vi "Disconnect All.vi"(8 "error in (no error)":errorcluster, 11 "Consumer in":refnum<class "Consumer.lvclass">) -> (0 "error out":errorcluster, 3 "Consumer out":refnum<class "Consumer.lvclass">)   [LabVIEW 2017, in "%DEVICE% Messaging.lvlib" / "Consumer.lvclass"]
uses:
  Consumer.lvclass
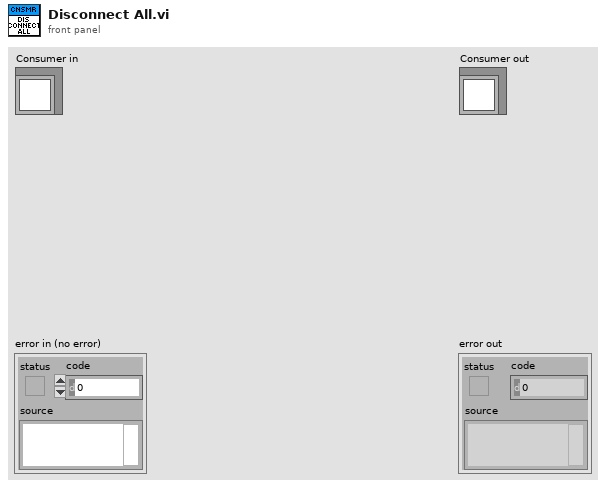
[diagram p1: front panel]
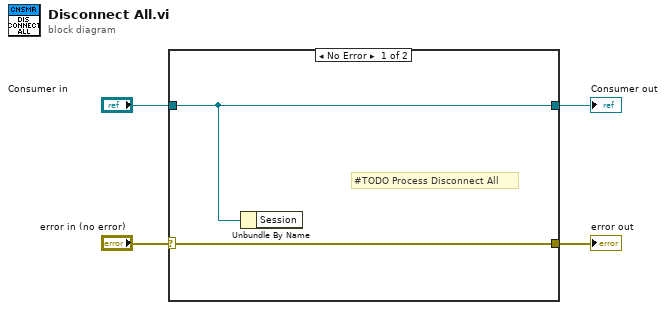
[diagram p0: block diagram]
diagram:
  n1 = case shown="No Error" "error in (no error)" {
    selector: "error in (no error)" -> [w5 w8]
    tunnel: [w5 w8] -> w3
    tunnel: [w6 w7] -> w1
    tunnel: "Consumer in" -> [w6 w7]
    frame No Error {
      # "#TODO Process Disconnect All"
      n2 = Unbundle By Name(w6) -> ()  [unwired: 1 out]
    }
    frame Error {
    }
  }
  "error out" <- w3
  "Consumer out" <- w1
